vi "WebSockets_Copy.vi"(0 "XRef":T5, 1 "State In":T1) -> (14 "Reply":T3, 15 "Fatal Error Out":T2, 16 "State Out":T1)   [LabVIEW 2020, in "WebSockets.xnode"]
doc: "Launches the JKI VI Package Manager (VIPM) where you can install the WebSockets Toolkit. The WebSockets Toolkit provides VIs for data streaming to/from web user interfaces, like WebVIs. \n\nAfter installing the toolkit, find the WebSockets VIs on the <b>Data Communication>>WebSockets</b> palette."
uses:
  <vilib>/WebSockets Toolkit/VIPMXNodeLink/WebSockets.xnode
  <vilib>/XNodeSupport/XNodeXNodeRef.ctl
  <vilib>/WebSockets Toolkit/VIPMXNodeLink/WebSockets.ctl
  <vilib>/XNodeSupport/XNodeStringArray.ctl
  <vilib>/XNodeSupport/XNodeString.ctl
  <vilib>/XNodeSupport/XNodeErrorCluster.ctl
  <vilib>/XNodeSupport/NI_XNodeSupport.lvlib
panel:
  in  "Error Message":string="Failed to launch the VI Package Manager. Please make sure you installed the VI Package Manager correctly."
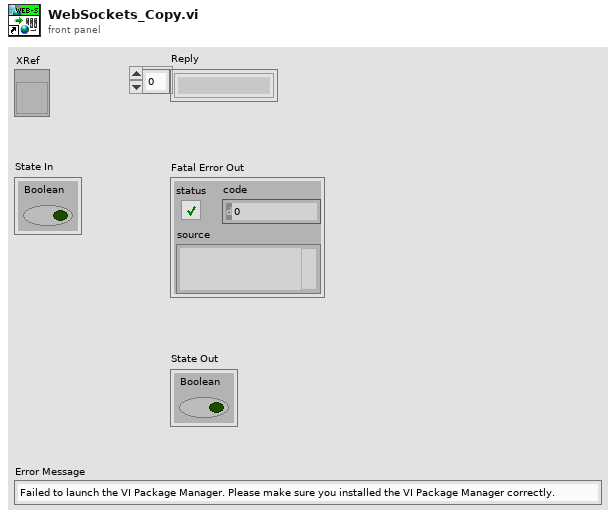
[diagram p1: front panel]
types:
  T1 = typedef "WebSockets.xnode/WebSockets.ctl" = cluster{"Boolean":bool}
  T2 = typedef "NI_XNodeSupport.lvlib/XNodeErrorCluster.ctl" = errorcluster
  T3 = typedef "NI_XNodeSupport.lvlib/XNodeStringArray.ctl" = T4[]
  T4 = typedef "NI_XNodeSupport.lvlib/XNodeString.ctl" = string
  T5 = typedef "NI_XNodeSupport.lvlib/XNodeXNodeRef.ctl" = refnum<vi>
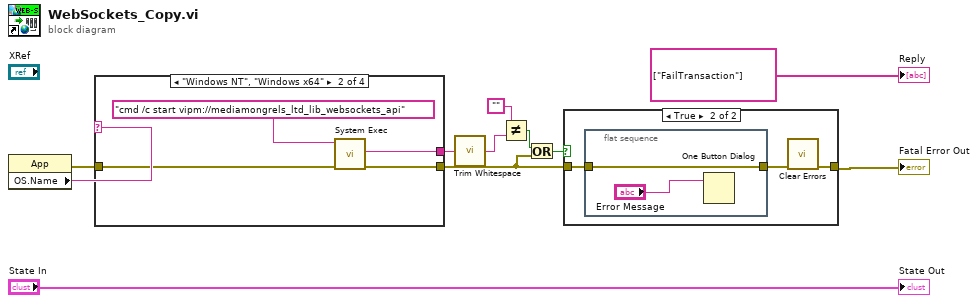
[diagram p0: block diagram]
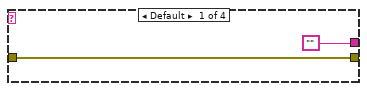
[diagram p2: hidden frame]
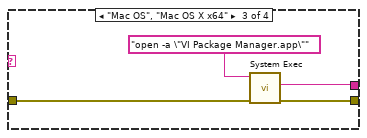
[diagram p3: hidden frame]
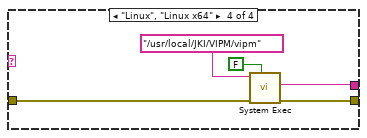
[diagram p4: hidden frame]
diagram:
  n1 = property class="App"() -> (error out=w3:errorcluster, "OS.Name"=w10:string)  [unwired: 2 in, 1 out]
  n2 = case shown="\"Windows NT\", \"Windows x64\"" w10 {
    tunnel: [w13 w17 w20 w24] -> w5
    tunnel: w3 -> [w13 w15 w21 w25]
    tunnel: ["" w14 w18 w23] -> w7
    frame Default {
    }
    frame "Windows NT", "Windows x64" {
      n3 = call <vilib>:"System Exec.vi"("error in (no error)"=w15, "command line"="cmd /c start vipm://mediamongrels_ltd_lib_websockets_api" ("URL")) -> ("error out"=w17:errorcluster, "standard error"=w14:string)  [unwired: 6 in, 2 out]
    }
    frame "Mac OS", "Mac OS X x64" {
      n4 = call <vilib>:"System Exec.vi"("error in (no error)"=w21, "command line"="open -a \"VI Package Manager.app\"" ("URL")) -> ("error out"=w20:errorcluster, "standard error"=w18:string)  [unwired: 6 in, 2 out]
    }
    frame "Linux", "Linux x64" {
      n5 = call <vilib>:"System Exec.vi"("wait until completion? (T)"=FALSE, "error in (no error)"=w25, "command line"="/usr/local/JKI/VIPM/vipm" ("URL")) -> ("error out"=w24:errorcluster, "standard error"=w23:string)  [unwired: 5 in, 2 out]
    }
  }
  n6 = call <vilib>:"Trim Whitespace.vi"("string"=w7) -> ("trimmed string"=w4:string)  [unwired: 1 in]
  n7 = Not Equal?(x="", y=w4) -> (x != y?=w8:bool)
  n8 = Or(x=w8, y=w5) -> (x .or. y?=w6:bool)
  n9 = case shown="True" w6 {
    tunnel: [w27 w30] -> w1
    tunnel: w5 -> [w27 w29]
    frame False {
    }
    frame True {
      n10 = flat-sequence {
        tunnel: w29 -> [w31]
        tunnel: [w31] -> w28
        frame #0 {
          n11 = One Button Dialog(message="Error Message") -> ()  [unwired: 1 in, 1 out]
        }
      }
      n12 = call <vilib>:"Clear Errors.vi"("error in (no error)"=w28) -> ("error out"=w30:errorcluster)  [unwired: 5 in, 1 out]
    }
  }
  "Fatal Error Out" <- w1
  "Reply" <- T3 ["FailTransaction"] ("Reply")
  "State Out" <- "State In"
